vi "GenerateCalTable.vi"(8 "CalFactorB":u8=10, 9 "CalFactorA":u8=10, 11 "DeviceType":u16) -> (3 "Array":dbl[][](array[numeric]))   [LabVIEW 2015]
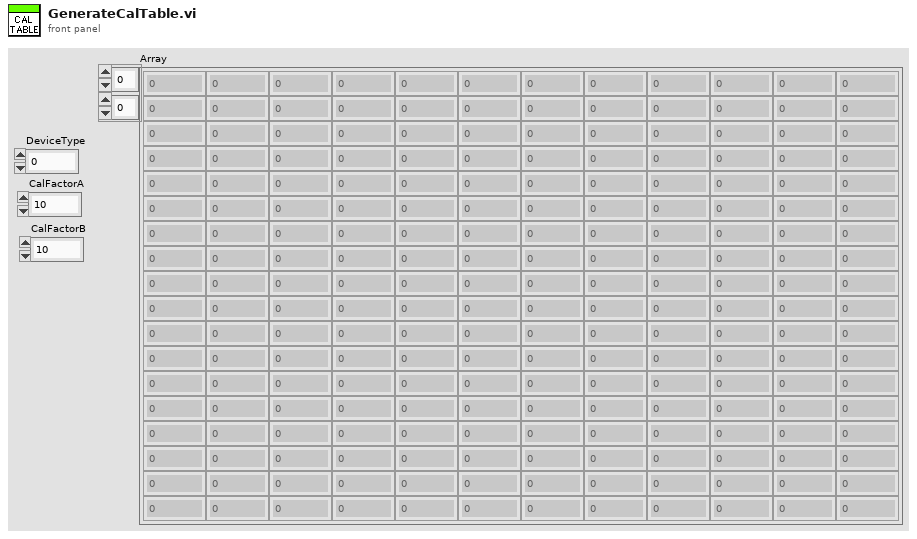
[diagram p1: front panel]
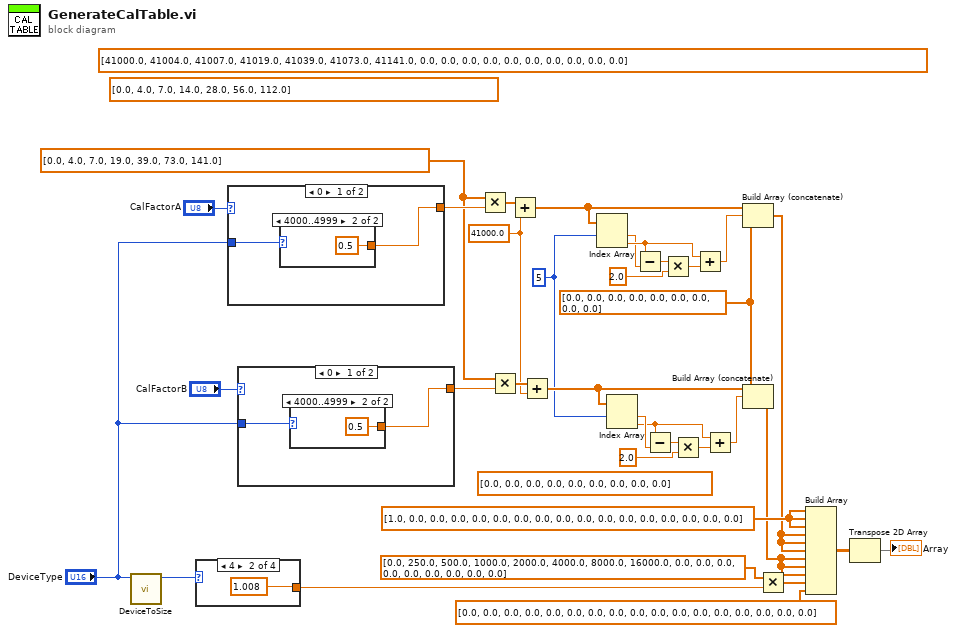
[diagram p0: block diagram]
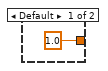
[diagram p2: hidden frame]
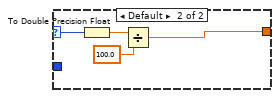
[diagram p3: hidden frame]
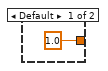
[diagram p4: hidden frame]
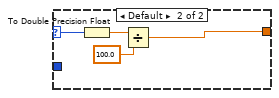
[diagram p5: hidden frame]
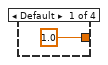
[diagram p6: hidden frame]
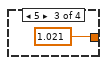
[diagram p7: hidden frame]
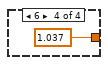
[diagram p8: hidden frame]
diagram:
  (unwired) dbl[] [0.0, 0.0, 0.0, 0.0, 0.0, 0.0, 0.0, 0.0, 0.0]
  w6 = dbl[] [0.0, 4.0, 7.0, 19.0, 39.0, 73.0, 141.0] ("Ref DataArr Out")
  w2 = 5 ("index")
  w5 = 41000.0
  w3 = dbl[] [0.0, 0.0, 0.0, 0.0, 0.0, 0.0, 0.0, 0.0, 0.0]
  (unwired) dbl[] [0.0, 4.0, 7.0, 14.0, 28.0, 56.0, 112.0] ("Ref DataArr Out")
  (unwired) dbl[] [41000.0, 41004.0, 41007.0, 41019.0, 41039.0, 41073.0, 41141.0, 0.0, 0.0, 0.0, 0.0, 0.0, 0.0, 0.0, 0.0, 0.0, 0.0] ("Ref DataArr Out")
  w32 = dbl[] [1.0, 0.0, 0.0, 0.0, 0.0, 0.0, 0.0, 0.0, 0.0, 0.0, 0.0, 0.0, 0.0, 0.0, 0.0, 0.0, 0.0] ("Ref DataArr Out")
  n1 = call "DeviceToSize.vi"("DeviceType in"="DeviceType") -> ("Size"=w18:u16)  [unwired: 9 in, 1 out]
  n2 = case shown="4" w18 {
    tunnel: [1.0 1.008 1.021 1.037] -> w1
    frame Default {
    }
    frame 4 {
    }
    frame 5 {
    }
    frame 6 {
    }
  }
  n3 = case shown="0" "CalFactorA" {
    selector: "CalFactorA" -> [_ w45]
    tunnel: [w40 w44] -> w19
    tunnel: "DeviceType" -> [w41 _]
    frame 0 {
      n4 = case shown="4000..4999" w41 {
        tunnel: [1.0 0.5] -> w40
        frame Default {
        }
        frame 4000..4999 {
        }
      }
    }
    frame Default {
      n5 = To Double Precision Float(number=w45) -> (double precision float=w46:dbl)
      n6 = Divide(x=w46, y=100.0) -> (x/y=w44:dbl)
    }
  }
  n7 = case shown="0" "CalFactorB" {
    selector: "CalFactorB" -> [_ w53]
    tunnel: [w48 w52] -> w17
    tunnel: "DeviceType" -> [w49 _]
    frame 0 {
      n8 = case shown="4000..4999" w49 {
        tunnel: [1.0 0.5] -> w48
        frame Default {
        }
        frame 4000..4999 {
        }
      }
    }
    frame Default {
      n9 = To Double Precision Float(number=w53) -> (double precision float=w54:dbl)
      n10 = Divide(x=w54, y=100.0) -> (x/y=w52:dbl)
    }
  }
  n11 = Multiply(x=w6, y=w19) -> (x*y=w29:dbl[])
  n12 = Multiply(x=w6, y=w17) -> (x*y=w9:dbl[])
  n13 = Add(x=w29, y=w5) -> (x+y=w22:dbl[])
  n14 = Add(x=w9, y=w5) -> (x+y=w15:dbl[])
  n15 = Index Array(array=w22, index #1=w2) -> (element #1=w23:dbl, element #2=w27:dbl)  [unwired: 1 in]
  n16 = Index Array(array=w15, index #1=w2) -> (element #1=w14:dbl, element #2=w10:dbl)  [unwired: 1 in]
  n17 = Subtract(x=w27, y=w23) -> (x-y=w24:dbl)
  n18 = Subtract(x=w10, y=w14) -> (x-y=w13:dbl)
  n19 = Multiply(x=w24, y=2.0) -> (x*y=w26:dbl)
  n20 = Multiply(x=w13, y=2.0) -> (x*y=w11:dbl)
  n21 = Add(x=w27, y=w26) -> (x+y=w21:dbl)
  n22 = Add(x=w10, y=w11) -> (x+y=w16:dbl)
  n23 = Build Array (concatenate)(w22, w21, w3) -> (w28:dbl[])
  n24 = Build Array (concatenate)(w15, w16, w3) -> (w4:dbl[])
  n25 = Multiply(x=dbl[] [0.0, 250.0, 500.0, 1000.0, 2000.0, 4000.0, 8000.0, 16000.0, 0.0, 0.0, 0.0, 0.0, 0.0, 0.0, 0.0, 0.0, 0.0] ("Ref DataArr Out"), y=w1) -> (x*y=w31:dbl[])
  n26 = Build Array(w32, w32, w32, w28, w28, w28, w4, w4, w4, w31, dbl[] [0.0, 0.0, 0.0, 0.0, 0.0, 0.0, 0.0, 0.0, 0.0, 0.0, 0.0, 0.0, 0.0, 0.0, 0.0, 0.0, 0.0] ("Ref DataArr Out")) -> (w35:dbl[][])
  n27 = Transpose 2D Array(2D array=w35) -> (transposed array=→"Array":dbl[][])
